vi "Read Stream and Create Channels.vi"(8 "error in (no error)":errorcluster, 10 "StreamReader Parameters in":T1, 11 "Plugin in":refnum<class "StreamReader.lvclass">) -> (0 "error out":errorcluster, 1 "Array":waveform(dbl)[](array[waveform]), 2 "StreamReader Parameters out":T1, 3 "Plugin out":refnum<class "StreamReader.lvclass">)   [LabVIEW 2024, in "StreamReader.lvlib" / "StreamReader.lvclass"]
uses:
  StreamReader.lvclass
  StreamReader Parameters.ctl
  <vilib>/FlexLogger/SDK/PluginSDK.lvlibp/PEFClasses/SDK/Producer Channel/Producer Channel.lvclass
  C:/Program Files/National Instruments/LabVIEW 2024/vi.lib/FlexLogger/SDK/PluginSDK.lvlibp/PEFClasses/SDK/Channel/Channel.lvclass
  StreamReader Strings.vi
  <vilib>/FlexLogger/SDK/PluginSDK.lvlibp/PEFClasses/SDK/Producer Channel/Create Producer Channel.vi
  StreamReader.lvclass/StreamReader.ctl
  <vilib>/FlexLogger/SDK/PluginSDK.lvlibp
  <resource>/objmgr/ni.dex.rc
  <vilib>/FlexLogger/SDK/PluginSDK.lvlibp/PEFClasses/SDK/Plugin/Plugin.lvclass
  C:/Program Files/National Instruments/LabVIEW 2024/vi.lib/FlexLogger/SDK/PluginSDK.lvlibp/PEFClasses/SDK/Plugin/Plugin.lvclass
  C:/Program Files/National Instruments/LabVIEW 2024/vi.lib/FlexLogger/SDK/PluginSDK.lvlibp/PEFClasses/SDK/Processing Element/Processing Element.lvclass
  C:/dev/niflexlogger-plugins/plugins/StreamReader/source/StreamReader/StreamReader.lvclass
  C:/Program Files/National Instruments/LabVIEW 2024/vi.lib/FlexLogger/SDK/PluginSDK.lvlibp/PEFClasses/SDK/Producer Channel/Producer Channel.lvclass
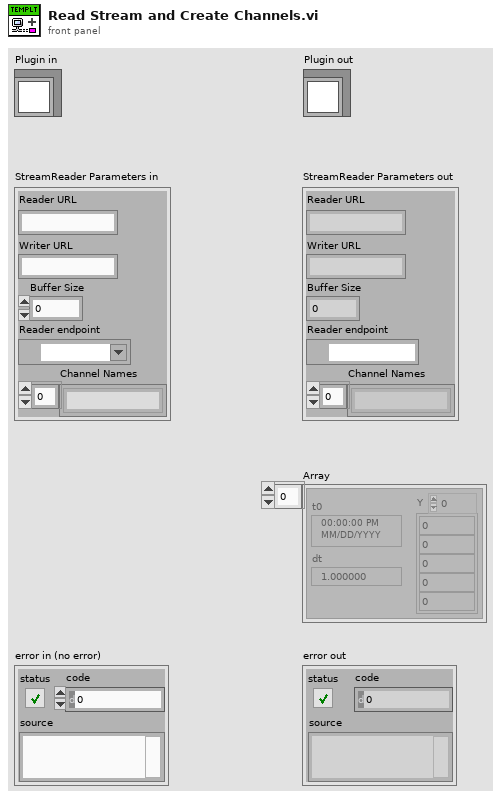
[diagram p1: front panel]
types:
  T1 = typedef "StreamReader.lvlib/StreamReader.lvclass/StreamReader Parameters.ctl" = cluster{"Reader URL":string, "Writer URL":string, "Buffer Size":i32, "Reader endpoint":refnum<k21>, "Channel Names":string[]}
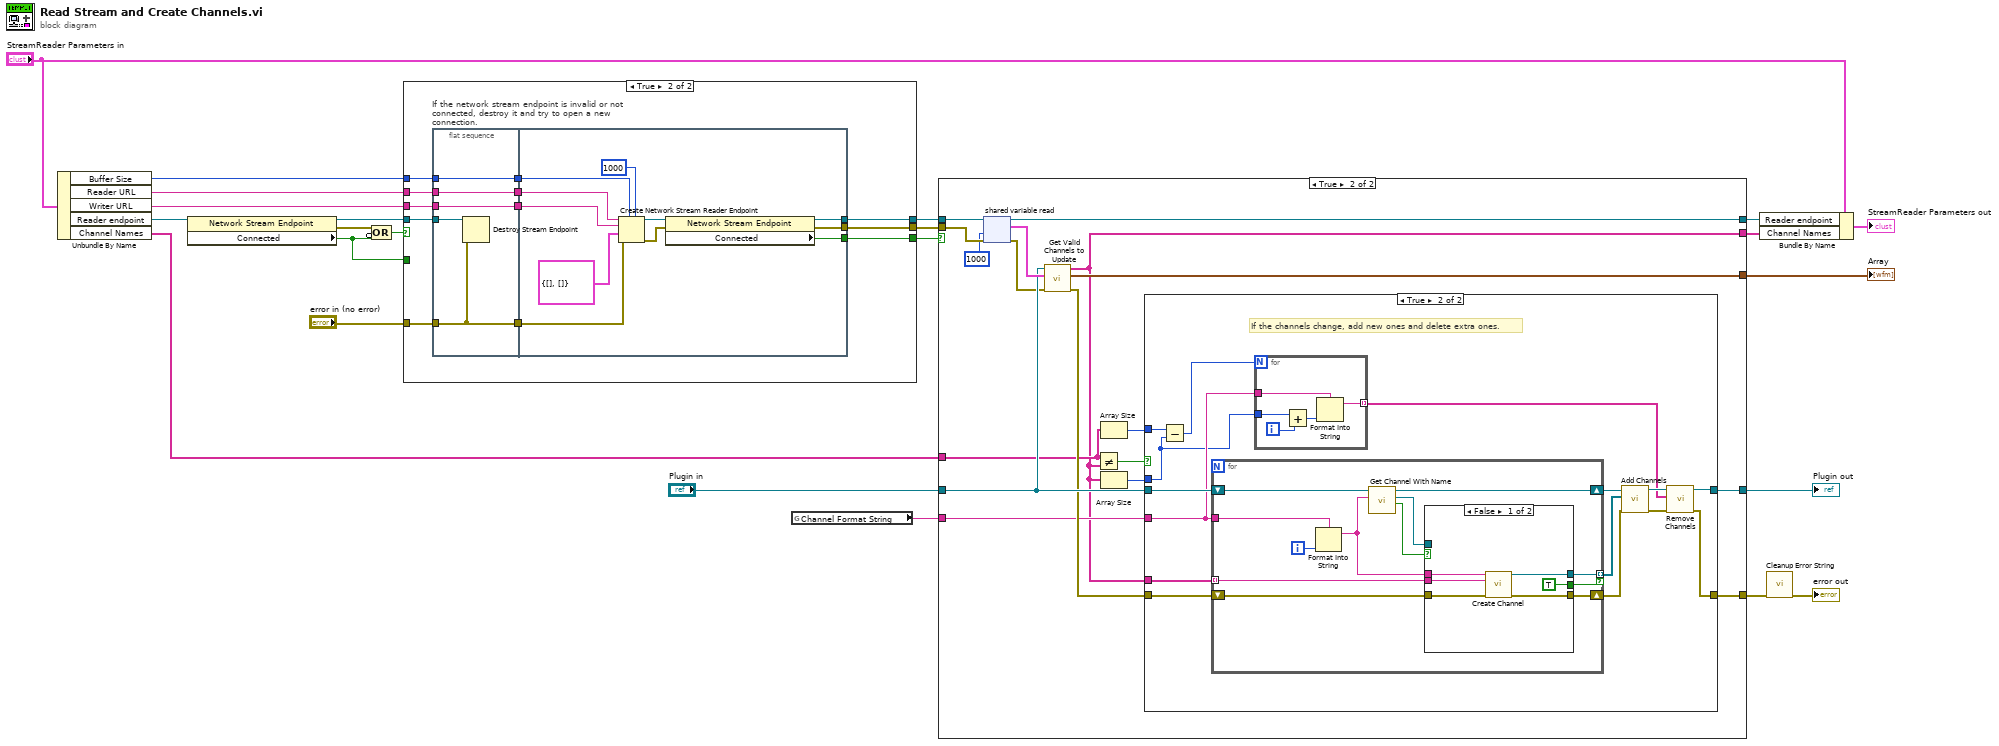
[diagram p0: block diagram]
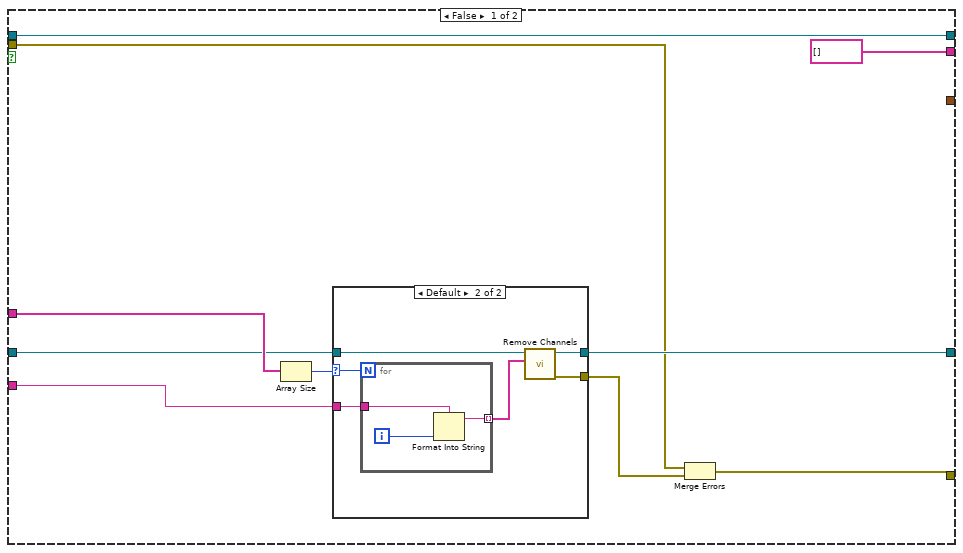
[diagram p3: hidden frame]
diagram:
  n1 = Unbundle By Name("StreamReader Parameters in") -> ("Buffer Size"=w18:i32, "Reader URL"=w19:string, "Writer URL"=w5:string, "Reader endpoint"=w17:refnum<k21>, "Channel Names"=w11:string[])
  n2 = property class="Network Stream Endpoint"(reference=w17) -> (reference out=w14:refnum<k21>, error out=w16:errorcluster, "Connected"=w13:bool)  [unwired: 1 in]
  n3 = Compound Arithmetic op=OR(w16, invert w13) -> (w15:bool)
  n4 = case shown="True" w15 {
    tunnel: [w24 w38] -> w23
    tunnel: [w26 w37] -> w22
    tunnel: [w25 w36] -> w21
    tunnel: "error in (no error)" -> [w24 w35]
    tunnel: w19 -> [_ w34]
    tunnel: w18 -> [_ w33]
    tunnel: w14 -> [w25 w29]
    tunnel: w13 -> [w26 _]
    tunnel: w5 -> [_ w28]
    frame False {
    }
    frame True {
      n5 = flat-sequence "If the network stream endpoint is invalid or not connected, destroy it and try to open a new connection." {
        tunnel: w33 -> [w42]
        tunnel: w34 -> [w43]
        tunnel: w35 -> [w40]
        tunnel: [w40] -> w32
        tunnel: [w43] -> w31
        tunnel: [w42] -> w30
        tunnel: w29 -> [w41]
        tunnel: w28 -> [w39]
        tunnel: [w39] -> w27
        tunnel: [w45] -> w38
        tunnel: [w44] -> w37
        tunnel: [w51] -> w36
        tunnel: w32 -> [w50]
        tunnel: w31 -> [w47]
        tunnel: w30 -> [w49]
        tunnel: w27 -> [w48]
        frame #0 {
          n6 = Destroy Stream Endpoint(8:w40, 11:w41) -> ()  [unwired: 1 out]
        }
        frame #1 {
          n7 = Create Network Stream Reader Endpoint(5:1000 ("timeout in ms (-1)"), 7:w49, 8:w50, 9:cluster{waveform(dbl)[], string[]} {[], []}, 10:w48, 11:w47) -> (0:w53:errorcluster, 3:w54:refnum<k21>)  [unwired: 1 in]
          n8 = property class="Network Stream Endpoint"(reference=w54, error in=w53) -> (reference out=w51:refnum<k21>, error out=w45:errorcluster, "Connected"=w44:bool)
        }
      }
    }
  }
  n9 = global read "StreamReader Strings.vi" "Channel Format String"() -> (w3:string)
  n10 = case shown="True" w22 {
    tunnel: w21 -> [w64 w91]
    tunnel: w23 -> [w56 w90]
    tunnel: [w55 w88] -> w2
    tunnel: [w64 w86] -> w8
    tunnel: "Plugin in" -> [w60 w84]
    tunnel: [w59 w89] -> w12
    tunnel: w11 -> [w62 w78]
    tunnel: [_ w87] -> w10
    tunnel: [string[] [] ("Channels Out") w77] -> w7
    tunnel: w3 -> [w63 w80]
    frame False {
      n11 = Array Size(array=w62) -> (size(s)=w58:i32)
      n12 = case shown="Default" w58 {
        selector: w58 -> [_ w66]
        tunnel: w63 -> [_ w70]
        tunnel: w60 -> [w65 w69]
        tunnel: [_ w68] -> w57
        tunnel: [w65 w67] -> w59
        frame 0 {
        }
        frame Default {
          n13 = for {
            N: w66 -> [_]
            tunnel: [w74] -> w71 mode=indexing
            tunnel: w70 -> [w73]
            i -> [w72]
            n14 = Format Into String(format string=w73, w72) -> (resulting string=w74:string)  [unwired: 2 in, 1 out]
          }
          n15 = call-dynamic "Remove Channels.vi"("Unique Channel Identifiers to Delete"=w71, "Plugin in"=w69) -> ("error out"=w68:errorcluster, "Plugin out"=w67:refnum<class "StreamReader.lvclass">)  [unwired: 8 in]
        }
      }
      n16 = Merge Errors(w56, w57) -> (w55:errorcluster)
    }
    frame True {
      n17 = shared-variable-read(w91, w90, 1000 ("timeout ms (-1)")) -> (w86:refnum<k21>, w83:errorcluster, w85:cluster{waveform(dbl)[], string[]})  [unwired: 1 out]
      n18 = call "Get Valid Channels to Update.vi"("error in (no error)"=w83, "Data Read"=w85, "Plugin in"=w84) -> ("error out"=w82:errorcluster, "Waveforms Out"=w87:waveform(dbl)[], "Channels Out"=w77:string[])  [unwired: 6 in]
      n19 = Not Equal?(x=w78, y=w77) -> (x != y?=w81:bool)
      n20 = Array Size(array=w78) -> (size(s)=w75:i32)
      n21 = Array Size(array=w77) -> (size(s)=w76:i32)
      n22 = case shown="True" w81 {
        tunnel: w82 -> [w93 w108]
        tunnel: [w93 w94] -> w88
        tunnel: w84 -> [w92 w107]
        tunnel: w77 -> [_ w106]
        tunnel: [w92 w96] -> w89
        tunnel: w80 -> [_ w103]
        tunnel: w76 -> [_ w102]
        tunnel: w75 -> [_ w105]
        frame False {
        }
        frame True {
          # "If the channels change, add new ones and delete extra ones."
          n23 = Subtract(x=w105, y=w102) -> (x-y=w104:i32)
          n24 = for {
            tunnel: w106 -> [w115] mode=indexing
            shift-right: [w124] -> w97
            shift-left: w108 -> [w125]
            tunnel: [w123] -> w98 mode=indexing if=w114
            shift-right: [w119] -> w99
            shift-left: w107 -> [w120]
            tunnel: w103 -> [w117]
            i -> [w121]
            n25 = Format Into String(format string=w117, w121) -> (resulting string=w118:string)  [unwired: 2 in, 1 out]
            n26 = call <vilib>:"Get Channel With Name.vi"("Name"=w118, "Plugin in"=w120) -> ("Found?"=w122:bool, "Channel"=w116:refnum<class "Channel.lvclass">, "Plugin out"=w119:refnum<class "StreamReader.lvclass">)  [unwired: 7 in]
            n27 = case shown="False" w122 {
              tunnel: w125 -> [w131 w132]
              tunnel: [w129 w132] -> w124
              tunnel: [w130 _] -> w123
              tunnel: w115 -> [w127 _]
              tunnel: w118 -> [w128 _]
              tunnel: w116 -> [_ _]
              tunnel: [TRUE _] -> w114
              frame False {
                n28 = call-poly <vilib>:"Create Channel.vi"("Unique Channel Identifier"=w128, "Default Channel Name"=w127, "error in (no error)"=w131) -> ("Producer Channel"=w130:refnum<class "Producer Channel.lvclass">, "error out"=w129:errorcluster)  [unwired: 11 in]
              }
              frame True {
              }
            }
          }
          n29 = for {
            N: w104 -> [_]
            tunnel: w102 -> [w113]
            tunnel: [w110] -> w95 mode=indexing
            tunnel: w103 -> [w109]
            i -> [w112]
            n30 = Add(x=w113, y=w112) -> (x+y=w111:i32)
            n31 = Format Into String(format string=w109, w111) -> (resulting string=w110:string)  [unwired: 2 in, 1 out]
          }
          n32 = call <vilib>:"Add Channels.vi"("error in (no error)"=w97, "Channels"=w98, "Plugin in"=w99) -> ("error out"=w101:errorcluster, "Plugin out"=w100:refnum<class "StreamReader.lvclass">)  [unwired: 7 in]
          n33 = call-dynamic "Remove Channels.vi"("error in (no error)"=w101, "Unique Channel Identifiers to Delete"=w95, "Plugin in"=w100) -> ("error out"=w94:errorcluster, "Plugin out"=w96:refnum<class "StreamReader.lvclass">)  [unwired: 7 in]
        }
      }
    }
  }
  "Plugin out" <- w12
  "Array" <- w10
  n34 = Bundle By Name(cluster="StreamReader Parameters in", "Reader endpoint"=w8, "Channel Names"=w7) -> (→"StreamReader Parameters out":T1)
  n35 = call "Cleanup Error String.vi"("error in (no error)"=w2) -> ("error out"=→"error out":errorcluster)  [unwired: 10 in]
